vi "Stop Module.vi"(6 "Timeout to Wait for Stop (s) (-1: no timeout)":dbl=-1.0, 8 "error in (no error)":errorcluster, 9 "Wait for Module to Stop? (F)":bool, 10 "Origin":string) -> (0 "error out":errorcluster)   [LabVIEW 2019, in "Logger.lvlib"]
doc: "Send the Stop request to the Module's Main.vi.\n\nIf <b>Wait for Module to Stop?</b> is TRUE, this VI will wait until the module main VI stops, and will timeout at the <b>Timeout to Wait for Stop</b> value. This value defaults to \"-1\", which means the VI will not timeout, and will always wait until the module main VI stops before completing execution.\n\nNote: The <b>Timeout to Wait for Stop</b> value is ignored if 'Wait for Module to Stop?' is set to FALSE.\n_____\nBased on Delacor QMH Project Template 4.0.0.47.\n_____\nBased on Delacor QMH Project Template 5.0.0.82."
uses:
  Logger.lvlib
  Stop Argument--cluster.ctl
  <vilib>/event_ctls.llb/usereventprio.ctl
panel:
  # "Note: The 'Timeout to Wait for Stop' value is ignored if 'Wait for Module to Stop?' is set to FALSE."
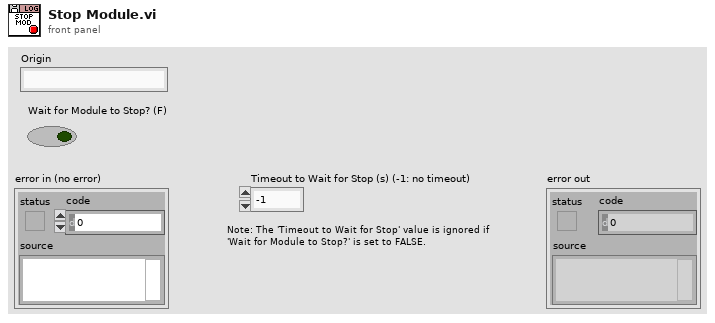
[diagram p1: front panel]
types:
  T1 = typedef "Logger.lvlib/Stop Argument--cluster.ctl" = cluster{"Origin":string, "Exit via Stop Module Req?":bool, "Wait for Module to stop?":bool}
  T2 = typedef "usereventprio.ctl" = enum32{"high priority", "normal priority"}
  T3 = typedef "Logger.lvlib/Request Events--cluster.ctl" = cluster{"Stop Module":refnum<user-event>, "Show Panel":refnum<user-event>, "Hide Panel":refnum<user-event>, "Get Module Execution Status":refnum<user-event>, "Show Diagram":refnum<user-event>, "Stop Logging":refnum<user-event>, "Log Data":refnum<user-event>, "Initialize File":refnum<user-event>}
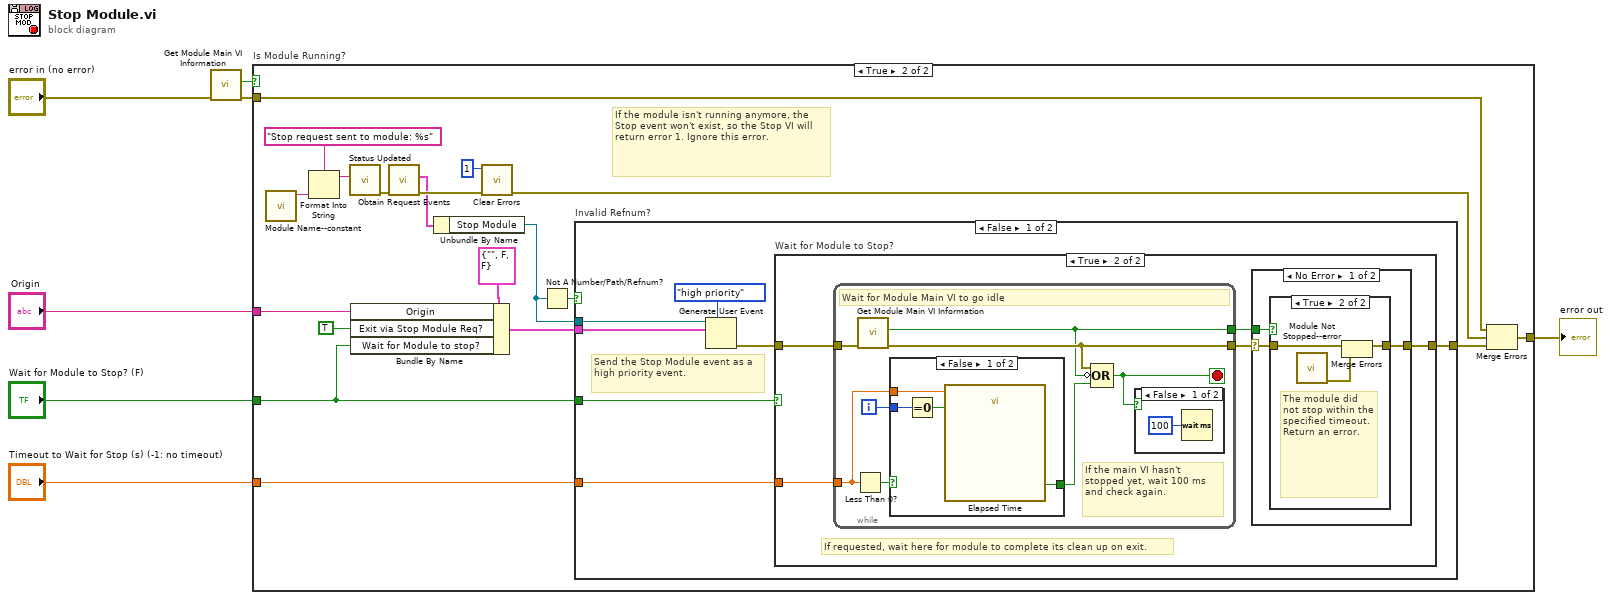
[diagram p0: block diagram]
diagram:
  n1 = call "Get Module Main VI Information.vi"("error in (no error)"="error in (no error)") -> ("error out"=w3:errorcluster, "Is Module Running?"=w2:bool)  [unwired: 7 in, 2 out]
  n2 = case "Is Module Running?" shown="True" w2 {
    tunnel: [w8 w26] -> w7
    tunnel: "Origin" -> [_ w25]
    tunnel: w3 -> [w8 w14]
    tunnel: "Wait for Module to Stop? (F)" -> [_ w10]
    tunnel: "Timeout to Wait for Stop (s) (-1: no timeout)" -> [_ w9]
    frame False {
      # "The module is not running, there is no need to run the Stop Module code."
    }
    frame True {
      # "If the module isn't running anymore, the Stop event won't exist, so the Stop VI will return error 1. Ignore this error."
      n3 = call "Module Name--constant.vi"() -> ("Module Name"=w21:string)  [unwired: 11 in]
      n4 = Format Into String(format string="Stop request sent to module: %s", w21) -> (resulting string=w22:string)  [unwired: 2 in, 1 out]
      n5 = call "Status Updated.vi"("Status"=w22) -> ("error out"=w13:errorcluster)  [unwired: 10 in]
      n6 = Bundle By Name(cluster=T1 {"Origin"="", "Exit via Stop Module Req?"=FALSE, "Wait for Module to stop?"=FALSE} ("event data"), "Origin"=w25, "Exit via Stop Module Req?"=TRUE, "Wait for Module to stop?"=w10) -> (w17:T1)
      n7 = call "Obtain Request Events.vi"("error in (no error)"=w13) -> ("error out"=w27:errorcluster, "Logger Request Events"=w24:T3)  [unwired: 9 in]
      n8 = Unbundle By Name(w24) -> ("Stop Module"=w18:refnum<user-event>)
      n9 = call <vilib>:"Clear Errors.vi"("error in (no error)"=w27, "specific error code to clear (0: all)"=1) -> ("error out"=w12:errorcluster)  [unwired: 4 in, 1 out]
      n10 = Not A Number/Path/Refnum?(number/path/refnum=w18) -> (NaN/Path/Refnum?=w19:bool)
      n11 = case "Invalid Refnum?" shown="False" w19 {
        tunnel: [w29 _] -> w16
        tunnel: w18 -> [w34 _]
        tunnel: w17 -> [w32 _]
        tunnel: w10 -> [w30 _]
        tunnel: w9 -> [w28 _]
        frame False {
          # "Send the Stop Module event as a high priority event."
          n12 = Generate User Event(priority (normal)=usereventprio."high priority", user event=w34, event data cluster=w32) -> (error out=w31:errorcluster)  [unwired: 1 in, 1 out]
          n13 = case "Wait for Module to Stop?" shown="True" w30 {
            tunnel: w31 -> [w35 w39]
            tunnel: [w35 w37] -> w29
            tunnel: w28 -> [_ w40]
            frame False {
            }
            frame True {
              # "If requested, wait here for module to complete its clean up on exit."
              n14 = while {
                tunnel: w40 -> [w51]
                tunnel: w39 -> [w55]
                tunnel: [w54] -> w38
                tunnel: [w53] -> w36
                i -> [w56]
                stop <- w49 stop-if-true
                # "If the main VI hasn't stopped yet, wait 100 ms and check again."
                # "Wait for Module Main VI to go idle"
                n15 = Less Than 0?(x=w51) -> (x < 0?=w50:bool)
                n16 = call "Get Module Main VI Information.vi"("error in (no error)"=w55) -> ("error out"=w54:errorcluster, "Is Module Running?"=w53:bool)  [unwired: 7 in, 2 out]
                n17 = case shown="False" w50 {
                  tunnel: w51 -> [w58 _]
                  tunnel: w56 -> [w60 _]
                  tunnel: [w59 _] -> w52
                  frame False {
                    n18 = Equal To 0?(x=w60) -> (x = 0?=w61:bool)
                    n19 = call "Elapsed Time"("Time Target (s)"=w58, "Reset"=w61) -> ("Time has Elapsed"=w59:bool)  [unwired: 10 in, 7 out]
                  }
                  frame True {
                    # "User specified a timeout of -1, so don't keep track of the elapsed time since this loop started."
                  }
                }
                n20 = Compound Arithmetic op=OR(w54, invert w53, w52) -> (w49:bool)
                n21 = case shown="False" w49 {
                  frame False {
                    n22 = Wait (ms)(milliseconds to wait=u32 100) -> ()  [unwired: 1 out]
                  }
                  frame True {
                  }
                }
              }
              n23 = case shown="No Error" w38 {
                selector: w38 -> [w42 w48]
                tunnel: [w41 w48] -> w37
                tunnel: w36 -> [w43 _]
                frame No Error {
                  n24 = case shown="True" w43 {
                    tunnel: w42 -> [w44 w47]
                    tunnel: [w44 w46] -> w41
                    frame False {
                      # "The module stopped, and no error occurred."
                    }
                    frame True {
                      # "The module did not stop within the specified timeout. Return an error."
                      n25 = call "Module Not Stopped--error.vi"() -> ("error out"=w45:errorcluster)  [unwired: 11 in]
                      n26 = Merge Errors(w47, w45) -> (w46:errorcluster)
                    }
                  }
                }
                frame Error {
                  # "An error occurred while waiting for the module to stop. Return that error."
                }
              }
            }
          }
        }
        frame True {
          # "Module is exiting. No need to send the standard \"not running\" error that is sent in other request VIs."
        }
      }
      n27 = Merge Errors(w14, w12, w16) -> (w26:errorcluster)
    }
  }
  "error out" <- w7
